vi "unpublish in mapping.vi"(7 "module ID":string, 8 "error in":errorcluster, 10 "published element":string, 11 "mappings in":T1) -> (0 "error out":errorcluster, 3 "mappings out":T1)   [LabVIEW 2013, in "engine configuration.lvclass"]
uses:
  engine configuration.lvclass
  simple mapping.ctl
  module channel pairings.ctl
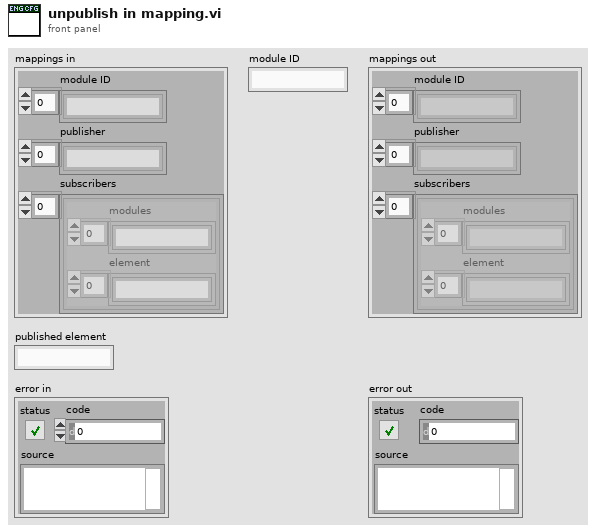
[diagram p1: front panel]
types:
  T1 = typedef "engine configuration.lvclass/simple mapping.ctl" = cluster{"module ID":string[], "publisher":string[], "subscribers":T2[]}
  T2 = typedef "engine configuration.lvclass/module channel pairings.ctl" = cluster{"modules":string[], "element":string[]}
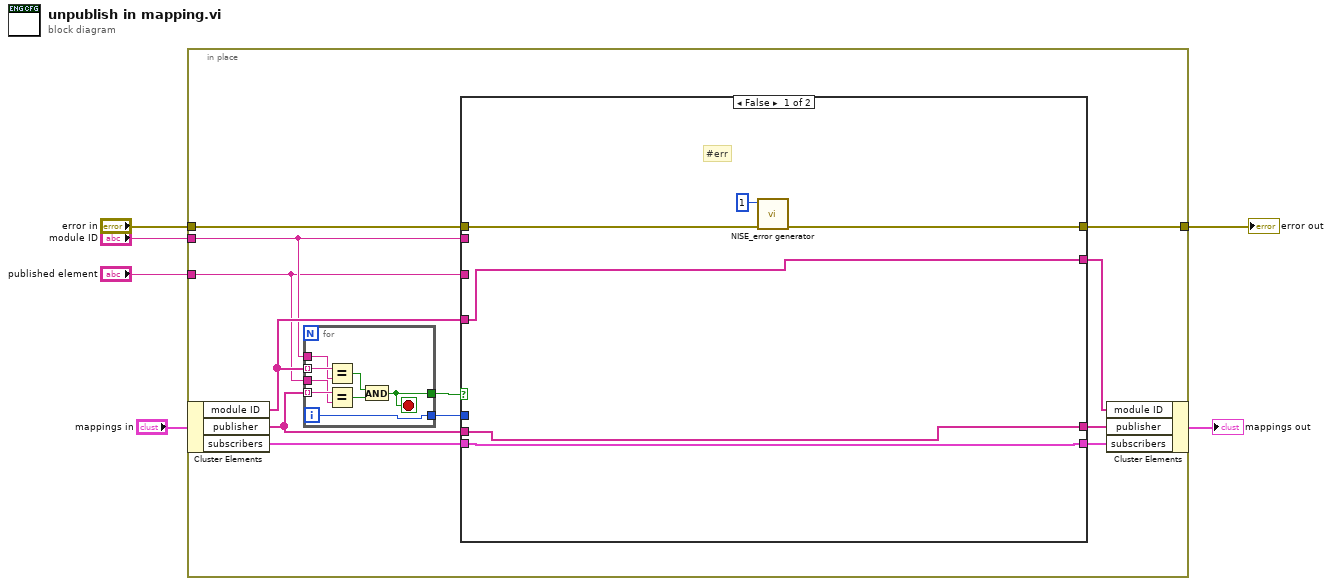
[diagram p0: block diagram]
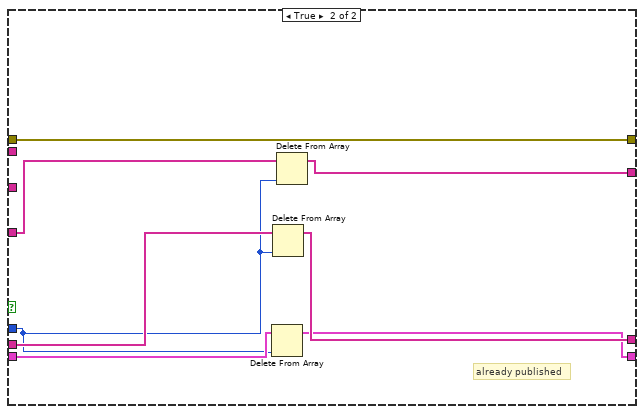
[diagram p2: hidden frame]
diagram:
  n1 = in-place {
    in-place-border: "module ID" -> [w9]
    in-place-border: "published element" -> [w8]
    in-place-border: [w11] -> w5
    in-place-border: "error in" -> [w10]
    n2 = in-place-cluster #1("mappings in") -> ("module ID"=w16:string[], "publisher"=w15:string[], "subscribers"=w12:T2[])
    n3 = for {
      tunnel: w16 -> [w40] mode=indexing
      tunnel: w15 -> [w39] mode=indexing
      tunnel: w9 -> [w38]
      tunnel: w8 -> [w37]
      tunnel: [w34] -> w18
      tunnel: [w33] -> w7
      i -> [w33]
      stop <- w34 stop-if-true
      n4 = Equal?(x=w40, y=w38) -> (x = y?=w35:bool)
      n5 = Equal?(x=w39, y=w37) -> (x = y?=w36:bool)
      n6 = And(x=w35, y=w36) -> (x .and. y?=w34:bool)
    }
    n7 = case shown="False" w18 {
      tunnel: [w21 w30] -> w17
      tunnel: w16 -> [w21 w31]
      tunnel: w15 -> [w22 w29]
      tunnel: [w22 w28] -> w14
      tunnel: [w23 w27] -> w13
      tunnel: w12 -> [w23 w26]
      tunnel: [w20 w32] -> w11
      tunnel: w10 -> [w24 w32]
      tunnel: w8 -> [_ _]
      tunnel: w9 -> [_ _]
      tunnel: w7 -> [_ w25]
      frame False {
        # "#err"
        n8 = call <vilib>:"NISE_error generator.vi"("error in"=w24, "error code (0)"=1) -> ("error out"=w20:errorcluster)  [unwired: 7 in]
      }
      frame True {
        # "already published"
        n9 = Delete From Array(array=w26, index=w25) -> (array with subset deleted=w27:T2[])  [unwired: 1 in, 1 out]
        n10 = Delete From Array(array=w29, index=w25) -> (array with subset deleted=w28:string[])  [unwired: 1 in, 1 out]
        n11 = Delete From Array(array=w31, index=w25) -> (array with subset deleted=w30:string[])  [unwired: 1 in, 1 out]
      }
    }
    n12 = in-place-cluster #1("module ID"=w17, "publisher"=w14, "subscribers"=w13) -> (→"mappings out":T1)
  }
  "error out" <- w5
